vi "reward_behavior_michelle_visjitter_conswinAdapt_enticefx_TSLog.vi"() -> ()   [LabVIEW 2019]
doc: "The myRIO Project template acquires acceleration data from the onboard accelerometer and displays the changes of acceleration values in a waveform chart."
uses:
  <vilib>/myRIO/Common/Instrument Driver Framework/Utilities/typedefs/Generic FPGA Reference.ctl
  <vilib>/myRIO/Common/Instrument Driver Framework/Utilities/typedefs/myRIO v1.0 Reference.ctl
  <vilib>/myRIO/Common/Instrument Driver Framework/Utilities/typedefs/Hardware Version Enum.ctl
  <vilib>/myRIO/Common/Instrument Driver Framework/Utilities/typedefs/myRIO Generic Hardware Reference.ctl
  <vilib>/userdefined/High Color/nirio_resource_hc.ctl
  <vilib>/myRIO/Common/Instrument Driver Framework/Utilities/vis/Is FPGA Ref Available.vi
  <vilib>/myRIO/Common/Instrument Driver Framework/myRIO v1.0/Encoder/typedefs/Encoder Signal Mode.ctl
  <vilib>/myRIO/Common/Instrument Driver Framework/myRIO v1.0/Encoder/typedefs/Encoder Channels Enum.ctl
  <vilib>/myRIO/Instrument Drivers/Onboard IO/Encoder/typedefs/Encoder Reference.ctl
  <vilib>/myRIO/Instrument Drivers/Onboard IO/Encoder/Encoder.lvlib
  <vilib>/myRIO/Instrument Drivers/Onboard IO/Encoder/vis/Read.vi
  <vilib>/myRIO/Common/Instrument Driver Framework/myRIO v1.0/Encoder/typedefs/Encoder Configuration v1.0.ctl
  <vilib>/myRIO/Common/Instrument Driver Framework/myRIO v1.0/Encoder/vis/myRIO v1.1 Open Encoder.vi
  <vilib>/myRIO/Common/Instrument Driver Framework/myRIO v1.0/Encoder/vis/myRIO v1.0 Configure Encoder.vi
  <vilib>/myRIO/Instrument Drivers/Onboard IO/Encoder/vis/myRIO Encoder Open.xnode
  <vilib>/myRIO/Express VI/Onboard IO/Encoder/Encoder Express VI.xnode
  <vilib>/myRIO/Express VI/Onboard IO/DI/DI Express VI.xnode
  <vilib>/myRIO/Instrument Drivers/Onboard IO/DIO/vis/Read.vi
  <vilib>/myRIO/Instrument Drivers/Onboard IO/DIO/DIO.lvlib
  <vilib>/myRIO/Common/Instrument Driver Framework/myRIO v1.0/DIO/typedefs/DIO Channels Enum.ctl
  <vilib>/myRIO/Common/Instrument Driver Framework/myRIO v1.0/DIO/typedefs/DIO Channels List.ctl
  <vilib>/myRIO/Instrument Drivers/Onboard IO/DIO/typedefs/DIO Reference.ctl
  <vilib>/myRIO/Instrument Drivers/Onboard IO/DIO/vis/myRIO DIO Open.xnode
  <vilib>/myRIO/Common/Instrument Driver Framework/myRIO v1.0/DIO/vis/myRIO v1.1 Open DIO.vi
  <vilib>/myRIO/Instrument Drivers/Onboard IO/DIO/vis/Write.vi
  <vilib>/myRIO/Express VI/Onboard IO/DO/DO Express VI.xnode
  <vilib>/Analysis/Matrix/Datatypes/RealMatrix.ctl
  <vilib>/Analysis/Matrix/NI_Matrix.lvlib
panel:
  out "EntTS":dbl[][](array[numeric])
  out "TimeLag":dbl
  out "Lag2":dbl
  out "TestTime":dbl
  out "RewTS":dbl[][](array[numeric])
  out "ConsTS":dbl[][](array[numeric])
  out "LickTS":dbl[][](array[numeric])
  out "ContrastChoice":dbl
  out "Its":i32
  out "BurstCriteria":dbl
  out "LickBurst 2":bool
  out "LickBurst":bool
  out "Enticements":i32
  in  "Entice":bool
  out "Misses":i32
  out "GoAhead":bool
  out "TimeOutDuration":i32
  out "ActiveTime":dbl
  out "ConsumptionGo":bool=TRUE
  out "Consumption_Period":i32
  out "Watch_Display":bool=TRUE
  in  "Give reward":bool
  out "Timings":dbl[](array[numeric])
  out "ISI":dbl
  out "ISI start time":dbl
  out "Time_out":bool=TRUE
  out "Time since lick":dbl
  out "Time of last lick":dbl
  out "Rewarded trials":dbl[](array[numeric])
  out "Rewards":u16
  out "Active Trial":bool
  out "Array temp2":T1
  out "Stimuli Loaded":bool
  out "Stim_ID":dbl[](array[numeric])
  out "Reward_mat":dbl[](array[numeric])
  out "Reward":bool=TRUE
  out "Frame clock":i32
  out "Licks":u32
  out "Lick":bool
  out "Time":dbl
  out "Stop":bool
  in  "Frames to collect":u32
  out "Overflow?":bool
  out "Counter Value":i32
  out "Velocity":dbl
  out "Velocity Plot":dbl[](graph)
  out "Velocity array":dbl[](array[numeric])
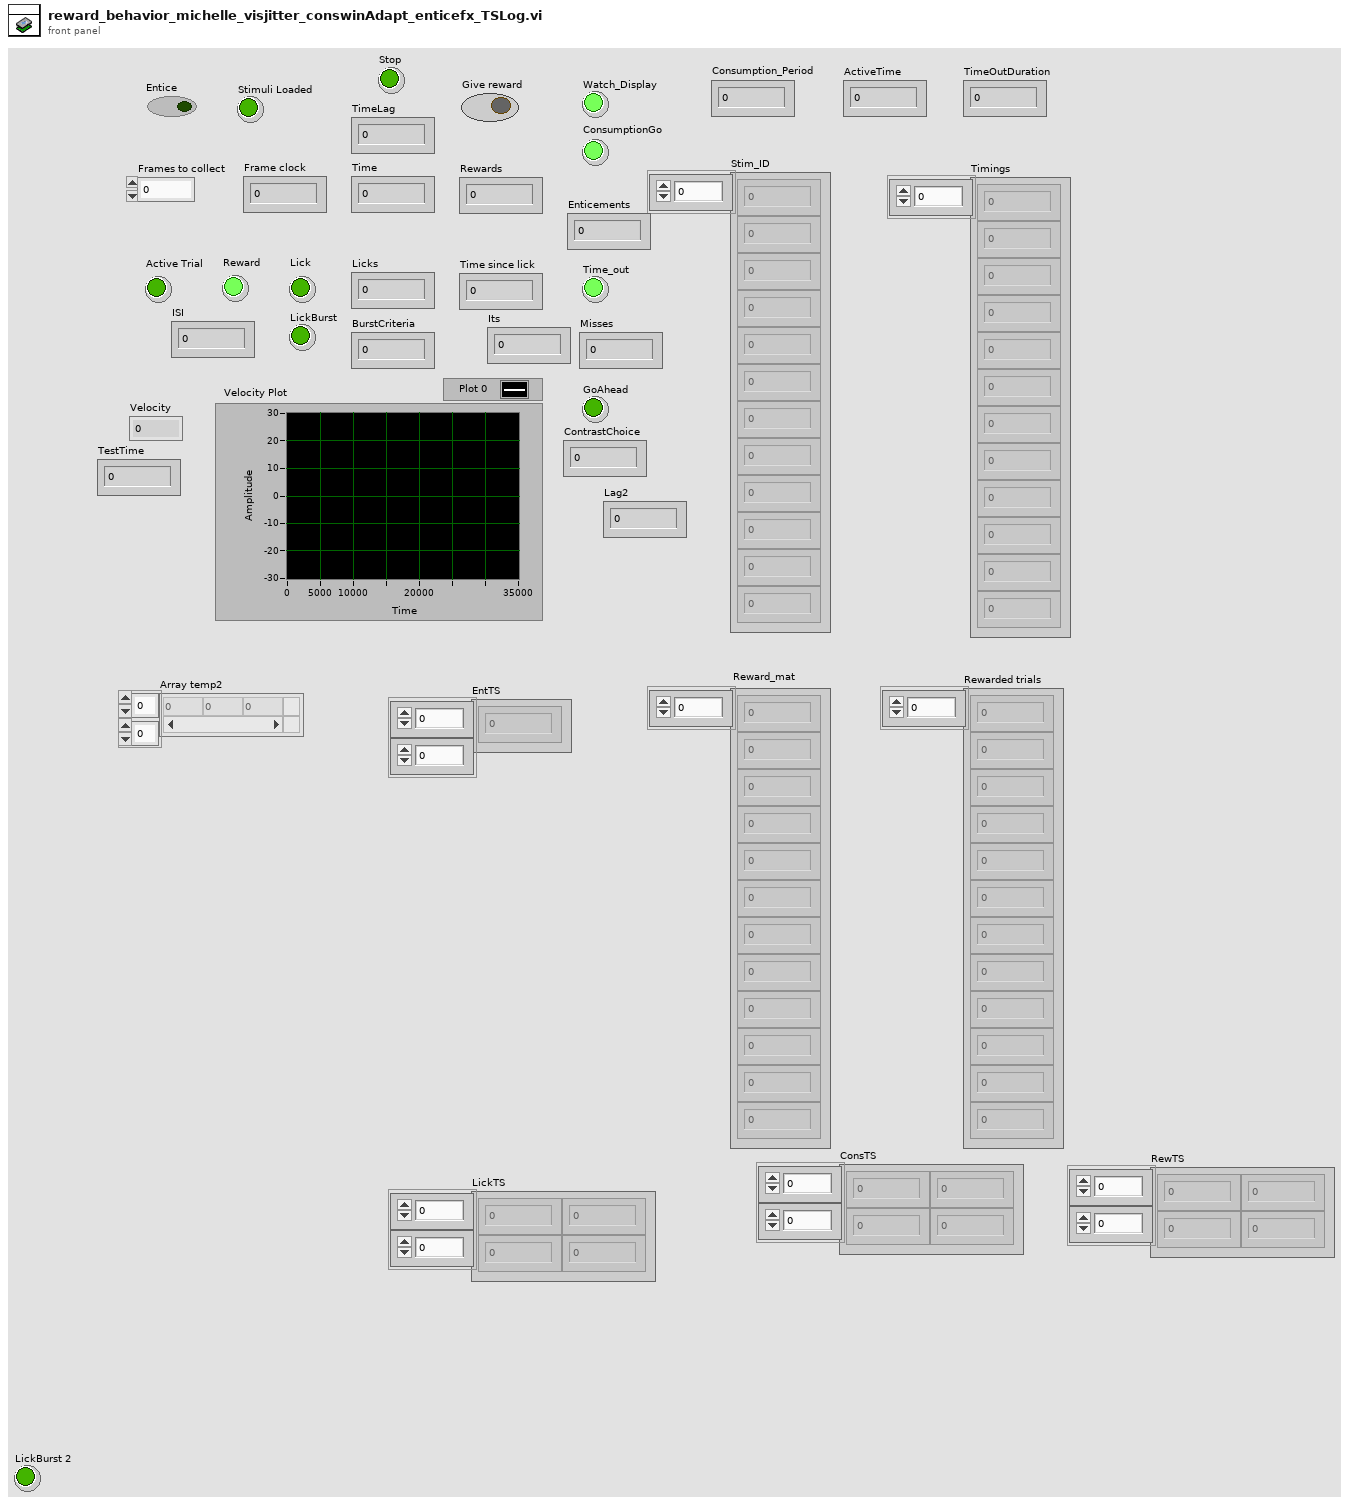
[diagram p1: front panel]
types:
  T1 = typedef "NI_Matrix.lvlib/RealMatrix.ctl" = dbl[][]
  T2 = typedef "Encoder.lvlib/Encoder Reference.ctl" = cluster{"myRIO Reference":T3, "Encoder Channels Enum":T7}
  T3 = typedef "myRIO Generic Hardware Reference.ctl" = cluster{"myRIO Model":T4, "myRIO Hardware Reference":T5}
  T4 = typedef "Hardware Version Enum.ctl" = enum16{"Unknown", "myRIO-1900", "myRIO-1950", "roboRIO", "NI ELVIS RIO CM", "ELVIS III"}
  T5 = typedef "myRIO v1.0 Reference.ctl" = cluster{"Generic FPGA Reference":T6, "Allow multiple opens":bool}
  T6 = typedef "Generic FPGA Reference.ctl" = refnum<k20>
  T7 = typedef "Encoder Channels Enum.ctl" = enum16{"Not Connected", "C/ENC0", "C/ENC1", "A/ENC", "A/ENC0", "A/ENC1", "A/ENC2", "A/ENC3", "A/ENC4", "A/ENC5", "A/ENC6", "A/ENC7", "A/ENC8", "A/ENC9", "B/ENC", "B/ENC0", "B/ENC1", "B/ENC2", "B/ENC3", "B/ENC4", "B/ENC5", "B/ENC6", "B/ENC7", "B/ENC8", "B/ENC9", "DIO/ENC0", "DIO/ENC1", "DIO/ENC2", "DIO/ENC3", "DIO/ENC4"}
  T8 = typedef "Encoder Signal Mode.ctl" = enum16{"Quadrature phase signal", "Step and direction signal"}
  T9 = typedef "nirio_resource_hc.ctl" = tag
  T10 = typedef "DIO.lvlib/DIO Reference.ctl" = cluster{"myRIO Reference":T3, "DIO Channels List":T11}
  T11 = typedef "DIO Channels List.ctl" = T12[]
  T12 = typedef "DIO Channels Enum.ctl" = enum16{"Not Connected", "C/DIO0", "C/DIO1", "C/DIO2", "C/DIO3", "C/DIO4", "C/DIO5", "C/DIO6", "C/DIO7", "A/DIO0", "A/DIO1", "A/DIO2", "A/DIO3", "A/DIO4", "A/DIO5", "A/DIO6", "A/DIO7", "A/DIO8", "A/DIO9", "A/DIO10", "A/DIO11", "A/DIO12", "A/DIO13", "A/DIO14", "A/DIO15", "A/DIO16", "A/DIO17", "A/DIO18", "A/DIO19", "B/DIO0", "B/DIO1", "B/DIO2", "B/DIO3", "B/DIO4", "B/DIO5", "B/DIO6", "B/DIO7", "B/DIO8", "B/DIO9", "B/DIO10", "B/DIO11", "B/DIO12", "B/DIO13", "B/DIO14", "B/DIO15", "B/DIO16", "B/DIO17", "B/DIO18", "B/DIO19", "LED0", "LED1", "LED2", "LED3", "Button0", "DIO/DIO0", "DIO/DIO1", "DIO/DIO2", "DIO/DIO3", "DIO/DIO4", "DIO/DIO5", "DIO/DIO6", "DIO/DIO7", "DIO/DIO8", "DIO/DIO9", "SPI/CS0", "SPI/CS1", "SPI/CS2", "SPI/CS3", "LED RADIO (Green)", "LED RADIO (Red)", "LED COMM (Green)", "LED COMM (Red)", "LED MODE (Green)", "LED MODE (Red)"}
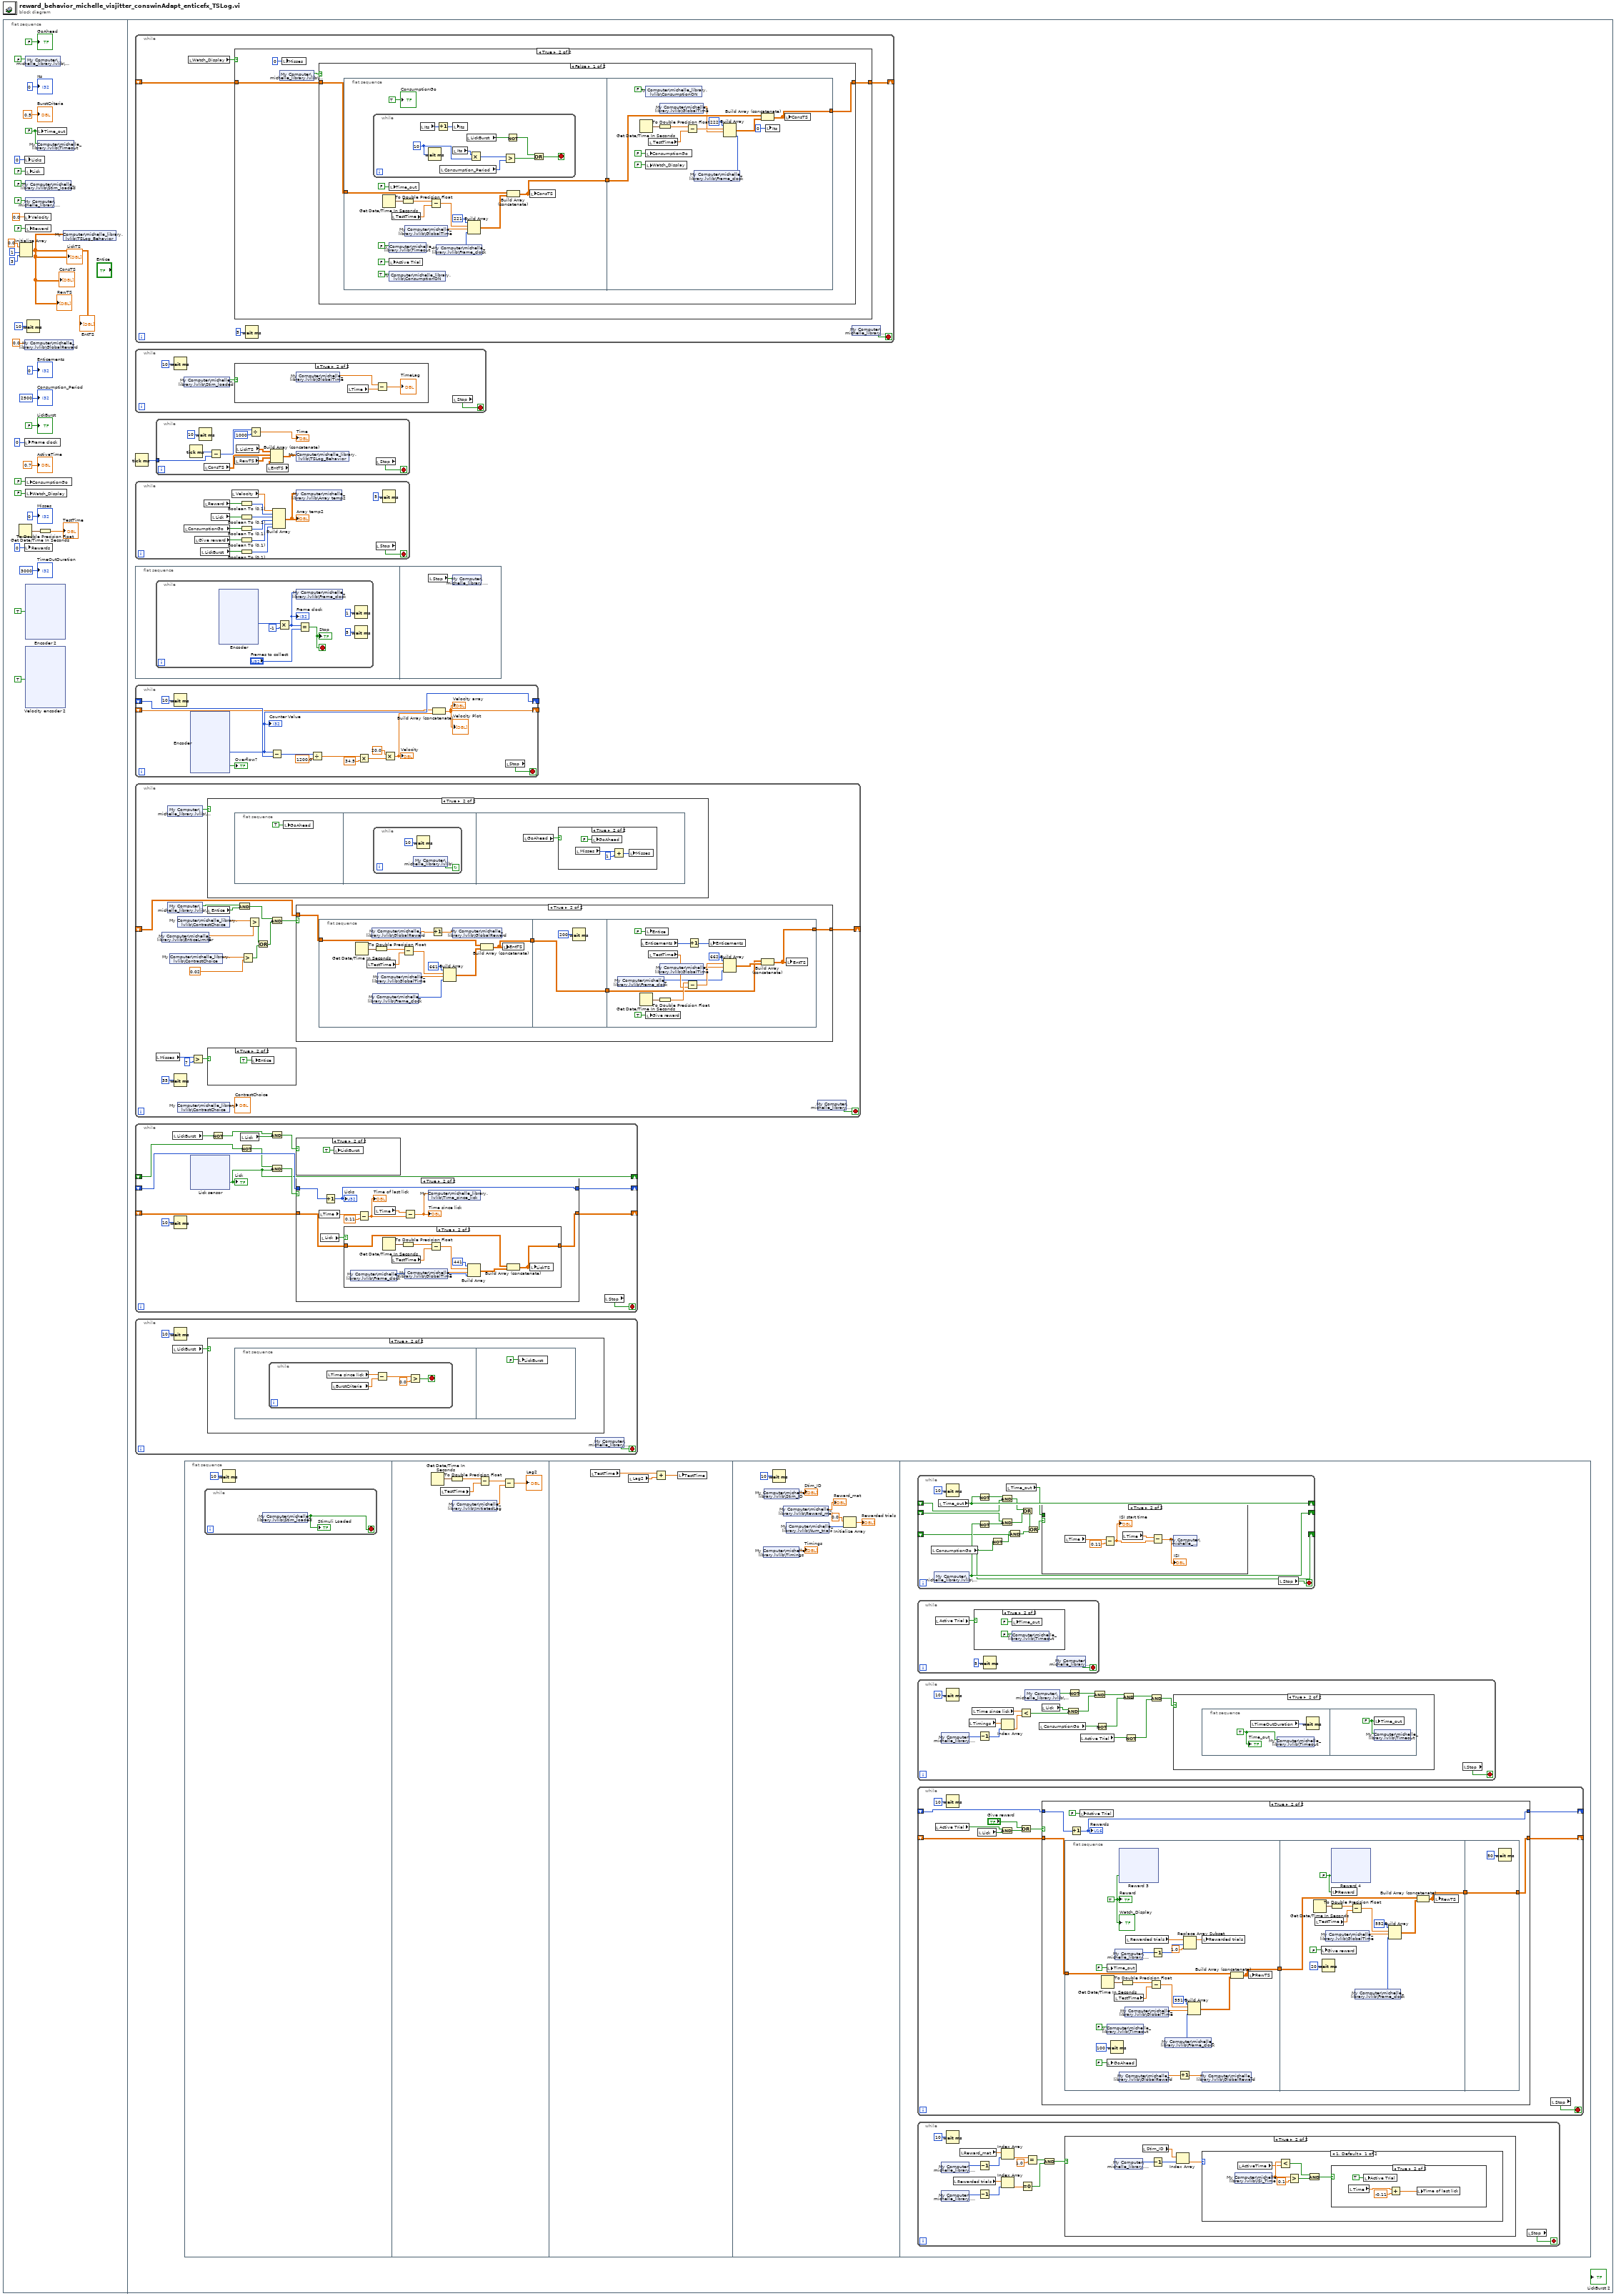
[diagram p0: block diagram]
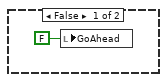
[diagram p6: hidden frame]
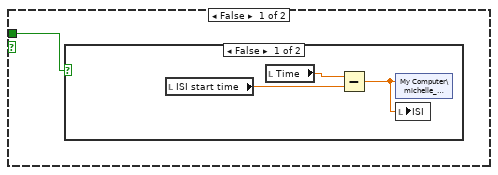
[diagram p12: hidden frame]
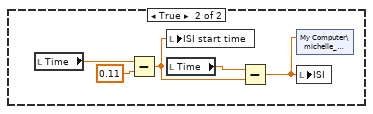
[diagram p13: hidden frame]
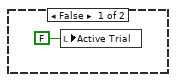
[diagram p14: hidden frame]
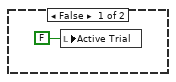
[diagram p15: hidden frame]
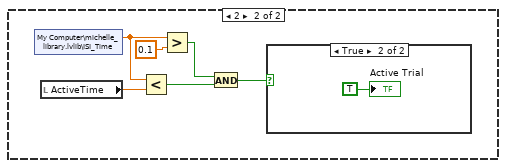
[diagram p16: hidden frame]
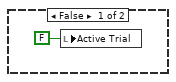
[diagram p17: hidden frame]
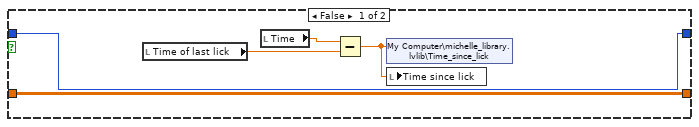
[diagram p20: hidden frame]
diagram:
  n1 = flat-sequence {
    frame #0 {
      w19 = FALSE ("Time_out")
      n2 = Get Date/Time In Seconds() -> (seconds since 1Jan1904=w3:timestamp)
      n3 = Initialize Array(0.0, 1, 3) -> (w1:dbl[][])
      "LickTS" <- w1
      "ConsTS" <- w1
      "RewTS" <- w1
      "EntTS" <- w1
      n4 = local write "Licks"(u32 0 ("Licks")) -> ()
      n5 = local write "Velocity"(0.0 ("Velocity")) -> ()
      n6 = shared-variable "My Computer\\michelle_library.lvlib\\GlobalReward"(0.0) -> ()  [unwired: 1 in, 1 out]
      n7 = local write "Frame clock"(u32 0 ("Frames")) -> ()
      n8 = local write "Rewards"(u16 0 ("Rewards")) -> ()
      n9 = shared-variable "My Computer\\michelle_library.lvlib\\Display"(FALSE ("Display")) -> ()  [unwired: 1 in, 1 out]
      n10 = local write "Lick"(FALSE ("Lick")) -> ()
      n11 = shared-variable "My Computer\\michelle_library.lvlib\\Stim_loaded"(FALSE ("Stim_loaded")) -> ()  [unwired: 1 in, 1 out]
      n12 = shared-variable "My Computer\\michelle_library.lvlib\\Stop"(FALSE ("Stop")) -> ()  [unwired: 1 in, 1 out]
      n13 = local write "Reward"(FALSE ("Give reward")) -> ()
      n14 = local write "ConsumptionGo"(FALSE ("ConsumptionGo")) -> ()
      n15 = local write "Watch_Display"(FALSE ("Watch_Display")) -> ()
      n16 = xnode "Encoder 2"("Reset Counter"=TRUE) -> ()  [unwired: 1 in, 4 out]
      n17 = xnode "Velocity encoder 2"("Reset Counter"=TRUE) -> ()  [unwired: 1 in, 4 out]
      n18 = Wait (ms)(milliseconds to wait=u32 10) -> ()  [unwired: 1 out]
      n19 = local write "Time_out"(w19) -> ()
      n20 = shared-variable "My Computer\\michelle_library.lvlib\\Timeout"(w19) -> ()  [unwired: 1 in, 1 out]
      n21 = To Double Precision Float(number=w3) -> (double precision float=→"TestTime":dbl)
      n22 = shared-variable "My Computer\\michelle_library.lvlib\\TSLog_Behavior"(w1) -> ()  [unwired: 1 in, 1 out]
      "Consumption_Period" <- 2500
      "ActiveTime" <- 0.7
      "TimeOutDuration" <- 3000
      "GoAhead" <- FALSE
      "Misses" <- 0
      "Enticements" <- 0
      "LickBurst" <- FALSE
      "BurstCriteria" <- 0.5
      "Its" <- 0
    }
    frame #1 {
      n23 = while {
        shift-right: [w203] -> _
        shift-left: _ -> [w204]
        stop <- w207 stop-if-true
        n24 = local read "Watch_Display"() -> (w206:bool)
        n25 = case shown="True" w206 {
          tunnel: w204 -> [w208 w210]
          tunnel: [w208 w209] -> w203
          frame False {
          }
          frame True {
            n26 = shared-variable "My Computer\\michelle_library.lvlib\\Display"() -> (w212:bool)  [unwired: 1 in, 1 out]
            n27 = local write "Misses"(0) -> ()
            n28 = case shown="False" w212 {
              tunnel: w210 -> [w215 w255]
              tunnel: [w213 w255] -> w209
              frame False {
                n29 = flat-sequence {
                  tunnel: w215 -> [w219]
                  tunnel: [w218] -> w214
                  tunnel: w214 -> [w245]
                  tunnel: [w244] -> w213
                  frame #0 {
                    n30 = while {
                      stop <- w234 stop-if-true
                      w235 = 10
                      n31 = local read "Its"() -> (w239:i32)
                      n32 = Wait (ms)(milliseconds to wait=w235) -> ()  [unwired: 1 out]
                      n33 = Increment(x=w239) -> (x+1=w238:i32)
                      n34 = local read "Consumption_Period"() -> (w232:i32)
                      n35 = local write "Its"(w238) -> ()
                      n36 = local read "Its"() -> (w236:i32)
                      n37 = local read "LickBurst"() -> (w240:bool)
                      n38 = Multiply(x=w236, y=w235) -> (x*y=w233:i32)
                      n39 = Greater?(x=w233, y=w232) -> (0:w231:bool)
                      n40 = Not(x=w240) -> (.not. x?=w237:bool)
                      n41 = Or(x=w237, y=w231) -> (x .or. y?=w234:bool)
                    }
                    n42 = Get Date/Time In Seconds() -> (seconds since 1Jan1904=w224:timestamp)
                    n43 = local write "Time_out"(FALSE) -> ()
                    n44 = shared-variable "My Computer\\michelle_library.lvlib\\Timeout"(FALSE) -> ()  [unwired: 1 in, 1 out]
                    n45 = local write "Active Trial"(FALSE) -> ()
                    n46 = shared-variable "My Computer\\michelle_library.lvlib\\ConsumptionON"(TRUE) -> ()  [unwired: 1 in, 1 out]
                    n47 = local read "TestTime"() -> (w221:dbl)
                    n48 = To Double Precision Float(number=w224) -> (double precision float=w222:dbl)
                    n49 = shared-variable "My Computer\\michelle_library.lvlib\\GlobalTime"() -> (w217:dbl)  [unwired: 1 in, 1 out]
                    n50 = Subtract(x=w222, y=w221) -> (x-y=w225:dbl)
                    n51 = shared-variable "My Computer\\michelle_library.lvlib\\Frame_clock"() -> (w216:u32)  [unwired: 1 in, 1 out]
                    n52 = Build Array(221, w225, w217, w216) -> (w220:T1)
                    n53 = Build Array (concatenate) ("Build Matrix")(w219, w220) -> (w218:T1)
                    n54 = local write "ConsTS"(w218) -> ()
                    "ConsumptionGo" <- TRUE
                  }
                  frame #1 {
                    n55 = Get Date/Time In Seconds() -> (seconds since 1Jan1904=w249:timestamp)
                    n56 = shared-variable "My Computer\\michelle_library.lvlib\\ConsumptionON"(FALSE) -> ()  [unwired: 1 in, 1 out]
                    n57 = local write "ConsumptionGo"(FALSE ("ConsumptionGo")) -> ()
                    n58 = local write "Watch_Display"(FALSE ("Watch_Display")) -> ()
                    n59 = local read "TestTime"() -> (w246:dbl)
                    n60 = To Double Precision Float(number=w249) -> (double precision float=w247:dbl)
                    n61 = shared-variable "My Computer\\michelle_library.lvlib\\GlobalTime"() -> (w242:dbl)  [unwired: 1 in, 1 out]
                    n62 = Subtract(x=w247, y=w246) -> (x-y=w250:dbl)
                    n63 = shared-variable "My Computer\\michelle_library.lvlib\\Frame_clock"() -> (w241:u32)  [unwired: 1 in, 1 out]
                    n64 = Build Array(222, w250, w242, w241) -> (w243:T1)
                    n65 = Build Array (concatenate) ("Build Matrix")(w245, w243) -> (w244:T1)
                    n66 = local write "Its"(0) -> ()
                    n67 = local write "ConsTS"(w244) -> ()
                  }
                }
              }
              frame True {
              }
            }
          }
        }
        n68 = Wait (ms)(milliseconds to wait=u32 5) -> ()  [unwired: 1 out]
        n69 = shared-variable "My Computer\\michelle_library.lvlib\\Stop"() -> (w207:bool)  [unwired: 1 in, 1 out]
      }
      n70 = while {
        stop <- w126 stop-if-true
        n71 = Wait (ms)(milliseconds to wait=u32 10) -> ()  [unwired: 1 out]
        n72 = shared-variable "My Computer\\michelle_library.lvlib\\Stim_loaded"() -> (w127:bool)  [unwired: 1 in, 1 out]
        n73 = case shown="True" w127 {
          frame False {
          }
          frame True {
            n74 = shared-variable "My Computer\\michelle_library.lvlib\\GlobalTime"() -> (w128:dbl)  [unwired: 1 in, 1 out]
            n75 = local read "Time"() -> (w129:dbl)
            n76 = Subtract(x=w128, y=w129) -> (x-y=→"TimeLag":dbl)
          }
        }
        n77 = local read "Stop"() -> (w126:bool)
      }
      n78 = Tick Count (ms)() -> (millisecond timer value=w124:u32)
      n79 = while {
        stop <- w263 stop-if-true
        n80 = local read "ConsumptionGo"() -> (w261:bool)
        n81 = local read "Give reward"() -> (w260:bool)
        n82 = local read "LickBurst"() -> (w257:bool)
        n83 = local read "Reward"() -> (w268:bool)
        n84 = local read "Lick"() -> (w269:bool)
        n85 = local read "Velocity"() -> (w267:dbl)
        n86 = Boolean To (0,1)(Boolean=w268) -> (0, 1=w266:i16)
        n87 = Boolean To (0,1)(Boolean=w269) -> (0, 1=w265:i16)
        n88 = Boolean To (0,1)(Boolean=w261) -> (0, 1=w259:i16)
        n89 = Boolean To (0,1)(Boolean=w260) -> (0, 1=w258:i16)
        n90 = Boolean To (0,1)(Boolean=w257) -> (0, 1=w256:i16)
        n91 = Build Array(w267, w266, w265, w259, w258, w256) -> (w262:T1)
        "Array temp2" <- w262
        n92 = shared-variable "My Computer\\michelle_library.lvlib\\Array temp2"(w262) -> ()  [unwired: 1 in, 1 out]
        n93 = local read "Stop"() -> (w263:bool)
        n94 = Wait (ms)(milliseconds to wait=u32 5) -> ()  [unwired: 1 out]
      }
      n95 = flat-sequence {
        frame #0 {
          n96 = while {
            stop <- w512 stop-if-true
            n97 = xnode "Encoder"() -> ("Counter Value"=w516:i32)  [unwired: 2 in, 3 out]
            n98 = Multiply(x=w516, y=-1) -> (x*y=w511:i32)
            "Frame clock" <- w511
            n99 = shared-variable "My Computer\\michelle_library.lvlib\\Frame_clock"(w511) -> ()  [unwired: 1 in, 1 out]
            n100 = Equal?(x=w511, y="Frames to collect") -> (x = y?=w512:bool)
            "Stop" <- w512
            n101 = Wait (ms)(milliseconds to wait=u32 1) -> ()  [unwired: 1 out]
            n102 = Wait (ms)(milliseconds to wait=u32 5) -> ()  [unwired: 1 out]
          }
        }
        frame #1 {
          n103 = local read "Stop"() -> (w564:bool)
          n104 = shared-variable "My Computer\\michelle_library.lvlib\\Stop"(w564) -> ()  [unwired: 1 in, 1 out]
        }
      }
      n105 = while {
        shift-right: [w651] -> _
        shift-left: _ -> [w652]
        shift-right: [w643] -> _
        shift-left: _ -> [w642]
        stop <- w641 stop-if-true
        n106 = Wait (ms)(milliseconds to wait=u32 10) -> ()  [unwired: 1 out]
        n107 = xnode "Encoder"() -> ("Counter Value"=w651:i32, "Overflow?"=→"Overflow?":bool)  [unwired: 2 in, 2 out]
        "Counter Value" <- w651
        n108 = Subtract(x=w651, y=w652) -> (x-y=w644:i32)
        n109 = Divide(x=w644, y=1200.0 ("600")) -> (x/y=w649:dbl)
        n110 = Multiply(x=w649, y=34.5) -> (x*y=w647:dbl)
        n111 = Multiply(x=20.0, y=w647) -> (x*y=w645:dbl)
        "Velocity" <- w645
        n112 = Build Array (concatenate)(w642, w645) -> (w643:dbl[])
        "Velocity Plot" <- w643
        "Velocity array" <- w643
        n113 = local read "Stop"() -> (w641:bool)
      }
      n114 = while {
        shift-right: [w146] -> _
        shift-left: _ -> [w147]
        stop <- w159 stop-if-true
        n115 = local read "Misses"() -> (w157:i32)
        n116 = shared-variable "My Computer\\michelle_library.lvlib\\EnticeLimiter"() -> (w145:dbl)  [unwired: 1 in, 1 out]
        n117 = shared-variable "My Computer\\michelle_library.lvlib\\Display"() -> (w158:bool)  [unwired: 1 in, 1 out]
        n118 = shared-variable "My Computer\\michelle_library.lvlib\\Display"() -> (w154:bool)  [unwired: 1 in, 1 out]
        n119 = shared-variable "My Computer\\michelle_library.lvlib\\ContrastChoice"() -> (w141:dbl)  [unwired: 1 in, 1 out]
        n120 = Wait (ms)(milliseconds to wait=35) -> ()  [unwired: 1 out]
        n121 = shared-variable "My Computer\\michelle_library.lvlib\\ContrastChoice"() -> (w150:dbl)  [unwired: 1 in, 1 out]
        n122 = shared-variable "My Computer\\michelle_library.lvlib\\ContrastChoice"() -> (→"ContrastChoice":dbl)  [unwired: 1 in, 1 out]
        n123 = Greater?(x=w157, y=7) -> (0:w155:bool)
        n124 = case shown="True" w158 {
          frame False {
            n125 = local write "GoAhead"(FALSE) -> ()
          }
          frame True {
            n126 = flat-sequence {
              frame #0 {
                n127 = local write "GoAhead"(TRUE) -> ()
              }
              frame #1 {
                n128 = while {
                  stop <- w197 continue-if-true
                  n129 = shared-variable "My Computer\\michelle_library.lvlib\\Display"() -> (w197:bool)  [unwired: 1 in, 1 out]
                  n130 = Wait (ms)(milliseconds to wait=10) -> ()  [unwired: 1 out]
                }
              }
              frame #2 {
                n131 = local read "GoAhead"() -> (w198:bool)
                n132 = case shown="True" w198 {
                  frame False {
                  }
                  frame True {
                    n133 = local read "Misses"() -> (w202:i32)
                    n134 = local write "GoAhead"(FALSE) -> ()
                    n135 = Add(x=w202, y=1) -> (x+y=w200:i32)
                    n136 = local write "Misses"(w200) -> ()
                  }
                }
              }
            }
          }
        }
        n137 = local read "Entice"() -> (w153:bool)
        n138 = case shown="True" w155 {
          frame False {
          }
          frame True {
            n139 = local write "Entice"(TRUE) -> ()
          }
        }
        n140 = And(x=w154, y=w153) -> (x .and. y?=w151:bool)
        n141 = Greater?(x=w141, y=0.02) -> (0:w142:bool)
        n142 = Greater?(x=w150, y=w145) -> (0:w143:bool)
        n143 = Or(x=w143, y=w142) -> (x .or. y?=w144:bool)
        n144 = And(x=w151, y=w144) -> (x .and. y?=w149:bool)
        n145 = case shown="True" w149 {
          tunnel: w147 -> [w160 w164]
          tunnel: [w160 w161] -> w146
          frame False {
          }
          frame True {
            n146 = flat-sequence {
              tunnel: w164 -> [w167]
              tunnel: [w166] -> w163
              tunnel: w163 -> [w177]
              tunnel: [w177] -> w162
              tunnel: w162 -> [w181]
              tunnel: [w180] -> w161
              frame #0 {
                n147 = Get Date/Time In Seconds() -> (seconds since 1Jan1904=w174:timestamp)
                n148 = local read "TestTime"() -> (w169:dbl)
                n149 = shared-variable "My Computer\\michelle_library.lvlib\\GlobalReward"() -> (w176:dbl)  [unwired: 1 in, 1 out]
                n150 = shared-variable "My Computer\\michelle_library.lvlib\\Frame_clock"() -> (w165:u32)  [unwired: 1 in, 1 out]
                n151 = To Double Precision Float(number=w174) -> (double precision float=w173:dbl)
                n152 = shared-variable "My Computer\\michelle_library.lvlib\\GlobalTime"() -> (w168:dbl)  [unwired: 1 in, 1 out]
                n153 = Subtract(x=w173, y=w169) -> (x-y=w172:dbl)
                n154 = Increment(x=w176) -> (x+1=w175:dbl)
                n155 = Build Array(661, w172, w168, w165) -> (w171:T1)
                n156 = shared-variable "My Computer\\michelle_library.lvlib\\GlobalReward"(w175) -> ()  [unwired: 1 in, 1 out]
                n157 = Build Array (concatenate) ("Build Matrix")(w167, w171) -> (w166:T1)
                n158 = local write "EntTS"(w166) -> ()
              }
              frame #1 {
                n159 = Wait (ms)(milliseconds to wait=200) -> ()  [unwired: 1 out]
              }
              frame #2 {
                n160 = shared-variable "My Computer\\michelle_library.lvlib\\Frame_clock"() -> (w179:u32)  [unwired: 1 in, 1 out]
                n161 = Get Date/Time In Seconds() -> (seconds since 1Jan1904=w188:timestamp)
                n162 = local read "Enticements"() -> (w190:i32)
                n163 = local write "Entice"(FALSE) -> ()
                n164 = local write "Give reward"(TRUE) -> ()
                n165 = local read "TestTime"() -> (w182:dbl)
                n166 = To Double Precision Float(number=w188) -> (double precision float=w187:dbl)
                n167 = shared-variable "My Computer\\michelle_library.lvlib\\GlobalTime"() -> (w183:dbl)  [unwired: 1 in, 1 out]
                n168 = Subtract(x=w187, y=w182) -> (x-y=w186:dbl)
                n169 = Increment(x=w190) -> (x+1=w189:i32)
                n170 = local write "Enticements"(w189) -> ()
                n171 = Build Array(662, w186, w183, w179) -> (w185:T1)
                n172 = Build Array (concatenate) ("Build Matrix")(w181, w185) -> (w180:T1)
                n173 = local write "EntTS"(w180) -> ()
              }
            }
          }
        }
        n174 = shared-variable "My Computer\\michelle_library.lvlib\\Stop"() -> (w159:bool)  [unwired: 1 in, 1 out]
      }
      n175 = while {
        shift-right: [w577] -> _
        shift-left: _ -> [w576]
        shift-right: [w571] -> _
        shift-left: _ -> [w574]
        shift-right: [w565] -> _
        shift-left: _ -> [w566]
        stop <- w575 stop-if-true
        n176 = local read "LickBurst"() -> (w568:bool)
        n177 = Wait (ms)(milliseconds to wait=u32 10) -> ()  [unwired: 1 out]
        n178 = xnode "Lick sensor"() -> ("C/DIO1 (DIO1)"=w571:bool)  [unwired: 1 in, 1 out]
        "Lick" <- w571
        n179 = Not(x=w568) -> (.not. x?=w567:bool)
        n180 = Not(x=w574) -> (.not. x?=w573:bool)
        n181 = local read "Lick"() -> (w569:bool)
        n182 = And(x=w567, y=w569) -> (x .and. y?=w570:bool)
        n183 = And(x=w573, y=w571) -> (x .and. y?=w572:bool)
        n184 = case shown="True" w570 {
          frame False {
          }
          frame True {
            n185 = local write "LickBurst"(TRUE) -> ()
          }
        }
        n186 = case shown="True" w572 {
          tunnel: [w584 w594] -> w577
          tunnel: w576 -> [w584 w593]
          tunnel: w566 -> [w580 w585]
          tunnel: [w580 w587] -> w565
          frame False {
            n187 = local read "Time of last lick"() -> (w582:dbl)
            n188 = local read "Time"() -> (w583:dbl)
            n189 = Subtract(x=w583, y=w582) -> (x-y=w581:dbl)
            n190 = shared-variable "My Computer\\michelle_library.lvlib\\Time_since_lick"(w581) -> ()  [unwired: 1 in, 1 out]
            n191 = local write "Time since lick"(w581) -> ()
          }
          frame True {
            n192 = local read "Time"() -> (w590:dbl)
            n193 = local read "Lick"() -> (w586:bool)
            n194 = Increment(x=w593) -> (x+1=w594:u32)
            "Licks" <- w594
            n195 = case shown="True" w586 {
              tunnel: w585 -> [w595 w601]
              tunnel: [w595 w600] -> w587
              frame False {
              }
              frame True {
                n196 = shared-variable "My Computer\\michelle_library.lvlib\\Frame_clock"() -> (w596:u32)  [unwired: 1 in, 1 out]
                n197 = Get Date/Time In Seconds() -> (seconds since 1Jan1904=w603:timestamp)
                n198 = local read "TestTime"() -> (w598:dbl)
                n199 = To Double Precision Float(number=w603) -> (double precision float=w599:dbl)
                n200 = shared-variable "My Computer\\michelle_library.lvlib\\GlobalTime"() -> (w597:dbl)  [unwired: 1 in, 1 out]
                n201 = Subtract(x=w599, y=w598) -> (x-y=w604:dbl)
                n202 = Build Array(441, w604, w597, w596) -> (w605:T1)
                n203 = Build Array (concatenate) ("Build Matrix")(w601, w605) -> (w600:T1)
                n204 = local write "LickTS"(w600) -> ()
              }
            }
            n205 = Subtract(x=w590, y=0.11) -> (x-y=w588:dbl)
            "Time of last lick" <- w588
            n206 = local read "Time"() -> (w592:dbl)
            n207 = Subtract(x=w592, y=w588) -> (x-y=w591:dbl)
            "Time since lick" <- w591
            n208 = shared-variable "My Computer\\michelle_library.lvlib\\Time_since_lick"(w591) -> ()  [unwired: 1 in, 1 out]
          }
        }
        n209 = local read "Stop"() -> (w575:bool)
      }
      n210 = while {
        stop <- w133 stop-if-true
        n211 = local read "LickBurst"() -> (w131:bool)
        n212 = Wait (ms)(milliseconds to wait=u32 10) -> ()  [unwired: 1 out]
        n213 = case shown="True" w131 {
          frame False {
          }
          frame True {
            n214 = flat-sequence {
              frame #0 {
                n215 = while {
                  stop <- w136 stop-if-true
                  n216 = local read "Time since lick"() -> (w137:dbl)
                  n217 = local read "BurstCriteria"() -> (w138:dbl)
                  n218 = Subtract(x=w137, y=w138) -> (x-y=w134:dbl)
                  n219 = Greater?(x=w134, y=0.0) -> (0:w136:bool)
                }
              }
              frame #1 {
                n220 = local write "LickBurst"(FALSE) -> ()
              }
            }
          }
        }
        n221 = shared-variable "My Computer\\michelle_library.lvlib\\Stop"() -> (w133:bool)  [unwired: 1 in, 1 out]
      }
      n222 = while {
        tunnel: w124 -> [w711]
        stop <- w709 stop-if-true
        n223 = Tick Count (ms)() -> (millisecond timer value=w712:u32)
        n224 = Wait (ms)(milliseconds to wait=u32 10) -> ()  [unwired: 1 out]
        n225 = local read "ConsTS"() -> (w704:dbl[][])
        n226 = Subtract(x=w712, y=w711) -> (x-y=w708:u32)
        n227 = local read "RewTS"() -> (w703:dbl[][])
        n228 = local read "LickTS"() -> (w705:dbl[][])
        n229 = Divide(x=w708, y=u32 1000) -> (x/y=→"Time":dbl)
        n230 = local read "EntTS"() -> (w701:dbl[][])
        n231 = Build Array (concatenate) ("Build Matrix")(w705, w704, w703, w701) -> (w702:T1)
        n232 = shared-variable "My Computer\\michelle_library.lvlib\\TSLog_Behavior"(w702) -> ()  [unwired: 1 in, 1 out]
        n233 = local read "Stop"() -> (w709:bool)
      }
      n234 = flat-sequence {
        frame #0 {
          n235 = while {
            stop <- w271 stop-if-true
            n236 = shared-variable "My Computer\\michelle_library.lvlib\\Stim_loaded"() -> (w271:bool)  [unwired: 1 in, 1 out]
            "Stimuli Loaded" <- w271
          }
          n237 = Wait (ms)(milliseconds to wait=u32 10) -> ()  [unwired: 1 out]
        }
        frame #1 {
          n238 = Get Date/Time In Seconds() -> (seconds since 1Jan1904=w277:timestamp)
          n239 = local read "TestTime"() -> (w276:dbl)
          n240 = To Double Precision Float(number=w277) -> (double precision float=w275:dbl)
          n241 = shared-variable "My Computer\\michelle_library.lvlib\\InitiatedLag"() -> (w274:dbl)  [unwired: 1 in, 1 out]
          n242 = Subtract(x=w275, y=w276) -> (x-y=w272:dbl)
          n243 = Subtract(x=w272, y=w274) -> (x-y=→"Lag2":dbl)
        }
        frame #2 {
          n244 = local read "TestTime"() -> (w278:dbl)
          n245 = local read "Lag2"() -> (w279:dbl)
          n246 = Add(x=w278, y=w279) -> (x+y=w280:dbl)
          n247 = local write "TestTime"(w280) -> ()
        }
        frame #3 {
          n248 = shared-variable "My Computer\\michelle_library.lvlib\\Timings"() -> (→"Timings":dbl[])  [unwired: 1 in, 1 out]
          n249 = shared-variable "My Computer\\michelle_library.lvlib\\Stim_ID"() -> (→"Stim_ID":dbl[])  [unwired: 1 in, 1 out]
          n250 = Wait (ms)(milliseconds to wait=u32 10) -> ()  [unwired: 1 out]
          n251 = shared-variable "My Computer\\michelle_library.lvlib\\Reward_mat"() -> (→"Reward_mat":dbl[])  [unwired: 1 in, 1 out]
          n252 = shared-variable "My Computer\\michelle_library.lvlib\\Num_trials"() -> (w284:u32)  [unwired: 1 in, 1 out]
          n253 = Initialize Array(0.0 ("element"), w284) -> (→"Rewarded trials":dbl[])
        }
        frame #4 {
          n254 = while {
            shift-right: [w330] -> _
            shift-left: _ -> [w328]
            shift-right: [w326] -> _
            shift-left: _ -> [w325]
            shift-right: [w320] -> _
            shift-left: _ -> [w318]
            stop <- w331 stop-if-true
            n255 = local read "ConsumptionGo"() -> (w320:bool)
            n256 = shared-variable "My Computer\\michelle_library.lvlib\\Display"() -> (w326:bool)  [unwired: 1 in, 1 out]
            n257 = local read "Time_out"() -> (w330:bool)
            n258 = Wait (ms)(milliseconds to wait=u32 10) -> ()  [unwired: 1 out]
            n259 = Not(x=w330) -> (.not. x?=w329:bool)
            n260 = Not(x=w326) -> (.not. x?=w324:bool)
            n261 = Not(x=w320) -> (.not. x?=w321:bool)
            n262 = And(x=w329, y=w328) -> (x .and. y?=w323:bool)
            n263 = And(x=w325, y=w324) -> (x .and. y?=w319:bool)
            n264 = local read "Time_out"() -> (w327:bool)
            n265 = And(x=w318, y=w321) -> (x .and. y?=w317:bool)
            n266 = Or(x=w323, y=w319) -> (x .or. y?=w316:bool)
            n267 = Or(x=w316, y=w317) -> (x .or. y?=w315:bool)
            n268 = case shown="True" w315 {
              tunnel: w327 -> [w332 _]
              frame False {
                n269 = case shown="False" w332 {
                  frame False {
                    n270 = local read "ISI start time"() -> (w335:dbl)
                    n271 = local read "Time"() -> (w334:dbl)
                    n272 = Subtract(x=w334, y=w335) -> (x-y=w333:dbl)
                    n273 = shared-variable "My Computer\\michelle_library.lvlib\\ISI"(w333) -> ()  [unwired: 1 in, 1 out]
                    n274 = local write "ISI"(w333) -> ()
                  }
                  frame True {
                    n275 = local read "Time"() -> (w340:dbl)
                    n276 = Subtract(x=w340, y=0.11) -> (x-y=w337:dbl)
                    n277 = local write "ISI start time"(w337) -> ()
                    n278 = local read "Time"() -> (w338:dbl)
                    n279 = Subtract(x=w338, y=w337) -> (x-y=w336:dbl)
                    n280 = shared-variable "My Computer\\michelle_library.lvlib\\ISI"(w336) -> ()  [unwired: 1 in, 1 out]
                    n281 = local write "ISI"(w336) -> ()
                  }
                }
              }
              frame True {
                n282 = local read "Time"() -> (w345:dbl)
                n283 = Subtract(x=w345, y=0.11) -> (x-y=w342:dbl)
                "ISI start time" <- w342
                n284 = local read "Time"() -> (w343:dbl)
                n285 = Subtract(x=w343, y=w342) -> (x-y=w341:dbl)
                "ISI" <- w341
                n286 = shared-variable "My Computer\\michelle_library.lvlib\\ISI"(w341) -> ()  [unwired: 1 in, 1 out]
              }
            }
            n287 = local read "Stop"() -> (w331:bool)
          }
          n288 = while {
            stop <- w290 stop-if-true
            n289 = local read "Active Trial"() -> (w289:bool)
            n290 = case shown="True" w289 {
              frame False {
              }
              frame True {
                n291 = local write "Time_out"(FALSE) -> ()
                n292 = shared-variable "My Computer\\michelle_library.lvlib\\Timeout"(FALSE) -> ()  [unwired: 1 in, 1 out]
              }
            }
            n293 = Wait (ms)(milliseconds to wait=5) -> ()  [unwired: 1 out]
            n294 = shared-variable "My Computer\\michelle_library.lvlib\\Stop"() -> (w290:bool)  [unwired: 1 in, 1 out]
          }
          n295 = while {
            stop <- w311 stop-if-true
            n296 = shared-variable "My Computer\\michelle_library.lvlib\\Trial"() -> (w301:u32)  [unwired: 1 in, 1 out]
            n297 = Wait (ms)(milliseconds to wait=u32 10) -> ()  [unwired: 1 out]
            n298 = local read "Timings"() -> (w303:dbl[])
            n299 = local read "Time since lick"() -> (w310:dbl)
            n300 = Decrement(x=w301) -> (x-1=w300:u32)
            n301 = Index Array(array=w303, index=w300) -> (element=w302:dbl)
            n302 = Less?(x=w310, y=w302) -> (x < y?=w309:bool)
            n303 = shared-variable "My Computer\\michelle_library.lvlib\\Display"() -> (w306:bool)  [unwired: 1 in, 1 out]
            n304 = local read "ConsumptionGo"() -> (w298:bool)
            n305 = local read "Lick"() -> (w308:bool)
            n306 = And(x=w308, y=w309) -> (x .and. y?=w304:bool)
            n307 = Not(x=w306) -> (.not. x?=w305:bool)
            n308 = local read "Active Trial"() -> (w293:bool)
            n309 = And(x=w305, y=w304) -> (x .and. y?=w297:bool)
            n310 = Not(x=w298) -> (.not. x?=w299:bool)
            n311 = And(x=w297, y=w299) -> (x .and. y?=w295:bool)
            n312 = Not(x=w293) -> (.not. x?=w296:bool)
            n313 = And(x=w295, y=w296) -> (x .and. y?=w294:bool)
            n314 = case shown="True" w294 {
              frame False {
              }
              frame True {
                n315 = flat-sequence {
                  frame #0 {
                    w313 = TRUE
                    n316 = local read "TimeOutDuration"() -> (w312:i32)
                    n317 = shared-variable "My Computer\\michelle_library.lvlib\\Timeout"(w313) -> ()  [unwired: 1 in, 1 out]
                    n318 = Wait (ms)(milliseconds to wait=w312) -> ()  [unwired: 1 out]
                    "Time_out" <- w313
                  }
                  frame #1 {
                    w314 = FALSE ("Timeout")
                    n319 = local write "Time_out"(w314) -> ()
                    n320 = shared-variable "My Computer\\michelle_library.lvlib\\Timeout"(w314) -> ()  [unwired: 1 in, 1 out]
                  }
                }
              }
            }
            n321 = local read "Stop"() -> (w311:bool)
          }
          n322 = while {
            shift-right: [w392] -> _
            shift-left: _ -> [w391]
            shift-right: [w384] -> _
            shift-left: _ -> [w385]
            stop <- w394 stop-if-true
            n323 = local read "Active Trial"() -> (w389:bool)
            n324 = Wait (ms)(milliseconds to wait=u32 10) -> ()  [unwired: 1 out]
            n325 = local read "Lick"() -> (w390:bool)
            n326 = And(x=w389, y=w390) -> (x .and. y?=w388:bool)
            n327 = Or(x="Give reward", y=w388) -> (x .or. y?=w387:bool)
            n328 = case shown="True" w387 {
              tunnel: [w396 w403] -> w392
              tunnel: w391 -> [w396 w402]
              tunnel: w385 -> [w395 w400]
              tunnel: [w395 w399] -> w384
              frame False {
              }
              frame True {
                n329 = flat-sequence {
                  tunnel: w400 -> [w409]
                  tunnel: [w406] -> w397
                  tunnel: [w465] -> w398
                  tunnel: w397 -> [w463]
                  tunnel: [w509] -> w399
                  tunnel: w398 -> [w509]
                  frame #0 {
                    w424 = TRUE ("C/DIO0 (DIO0)")
                    n330 = Get Date/Time In Seconds() -> (seconds since 1Jan1904=w413:timestamp)
                    n331 = local write "Time_out"(FALSE) -> ()
                    n332 = shared-variable "My Computer\\michelle_library.lvlib\\Timeout"(FALSE) -> ()  [unwired: 1 in, 1 out]
                    n333 = local write "GoAhead"(FALSE) -> ()
                    n334 = Wait (ms)(milliseconds to wait=u32 100) -> ()  [unwired: 1 out]
                    n335 = local read "TestTime"() -> (w407:dbl)
                    n336 = shared-variable "My Computer\\michelle_library.lvlib\\Trial"() -> (w423:u32)  [unwired: 1 in, 1 out]
                    n337 = xnode "Reward 3"("C/DIO0 (DIO0)"=w424) -> ()  [unwired: 1 in, 1 out]
                    n338 = shared-variable "My Computer\\michelle_library.lvlib\\GlobalReward"() -> (w415:dbl)  [unwired: 1 in, 1 out]
                    n339 = To Double Precision Float(number=w413) -> (double precision float=w412:dbl)
                    n340 = shared-variable "My Computer\\michelle_library.lvlib\\GlobalTime"() -> (w405:dbl)  [unwired: 1 in, 1 out]
                    n341 = local read "Rewarded trials"() -> (w421:dbl[])
                    n342 = Subtract(x=w412, y=w407) -> (x-y=w411:dbl)
                    n343 = Decrement(x=w423) -> (x-1=w422:u32)
                    n344 = shared-variable "My Computer\\michelle_library.lvlib\\Frame_clock"() -> (w404:u32)  [unwired: 1 in, 1 out]
                    n345 = Increment(x=w415) -> (x+1=w414:dbl)
                    n346 = Replace Array Subset(array=w421, new element=1.0 ("new element/subarray"), index=w422) -> (w419:dbl[])
                    n347 = Build Array(551, w411, w405, w404) -> (w410:T1)
                    n348 = local write "Rewarded trials"(w419) -> ()
                    n349 = shared-variable "My Computer\\michelle_library.lvlib\\GlobalReward"(w414) -> ()  [unwired: 1 in, 1 out]
                    n350 = Build Array (concatenate) ("Build Matrix")(w409, w410) -> (w406:T1)
                    n351 = local write "RewTS"(w406) -> ()
                    "Reward" <- w424
                    "Watch_Display" <- w424
                  }
                  frame #1 {
                    w473 = FALSE ("C/DIO0 (DIO0)")
                    n352 = Get Date/Time In Seconds() -> (seconds since 1Jan1904=w470:timestamp)
                    n353 = local read "TestTime"() -> (w464:dbl)
                    n354 = local write "Give reward"(FALSE ("Give reward")) -> ()
                    n355 = Wait (ms)(milliseconds to wait=u32 20) -> ()  [unwired: 1 out]
                    n356 = shared-variable "My Computer\\michelle_library.lvlib\\GlobalTime"() -> (w462:dbl)  [unwired: 1 in, 1 out]
                    n357 = To Double Precision Float(number=w470) -> (double precision float=w469:dbl)
                    n358 = xnode "Reward 4"("C/DIO0 (DIO0)"=w473) -> ()  [unwired: 1 in, 1 out]
                    n359 = local write "Reward"(w473) -> ()
                    n360 = Subtract(x=w469, y=w464) -> (x-y=w468:dbl)
                    n361 = shared-variable "My Computer\\michelle_library.lvlib\\Frame_clock"() -> (w461:u32)  [unwired: 1 in, 1 out]
                    n362 = Build Array(552, w468, w462, w461) -> (w466:T1)
                    n363 = Build Array (concatenate) ("Build Matrix")(w463, w466) -> (w465:T1)
                    n364 = local write "RewTS"(w465) -> ()
                  }
                  frame #2 {
                    n365 = Wait (ms)(milliseconds to wait=u32 50) -> ()  [unwired: 1 out]
                  }
                }
                n366 = Increment(x=w402) -> (x+1=w403:u16)
                "Rewards" <- w403
                n367 = local write "Active Trial"(FALSE ("Active Trial")) -> ()
              }
            }
            n368 = local read "Stop"() -> (w394:bool)
          }
          n369 = while {
            stop <- w359 stop-if-true
            n370 = shared-variable "My Computer\\michelle_library.lvlib\\Trial"() -> (w355:u32)  [unwired: 1 in, 1 out]
            n371 = shared-variable "My Computer\\michelle_library.lvlib\\Trial"() -> (w351:u32)  [unwired: 1 in, 1 out]
            n372 = Wait (ms)(milliseconds to wait=u32 10) -> ()  [unwired: 1 out]
            n373 = local read "Rewarded trials"() -> (w352:dbl[])
            n374 = local read "Reward_mat"() -> (w354:dbl[])
            n375 = Decrement(x=w355) -> (x-1=w356:u32)
            n376 = Decrement(x=w351) -> (x-1=w350:u32)
            n377 = Index Array(array=w354, index=w356) -> (element=w357:dbl)
            n378 = Index Array(array=w352, index=w350) -> (element=w349:dbl)
            n379 = Equal To 0?(x=w349) -> (x = 0?=w348:bool)
            n380 = Equal?(x=w357, y=1.0) -> (x = y?=w347:bool)
            n381 = And(x=w347, y=w348) -> (x .and. y?=w346:bool)
            n382 = case shown="True" w346 {
              frame False {
                n383 = local write "Active Trial"(FALSE ("Active_trial")) -> ()
              }
              frame True {
                n384 = shared-variable "My Computer\\michelle_library.lvlib\\Trial"() -> (w362:u32)  [unwired: 1 in, 1 out]
                n385 = local read "Stim_ID"() -> (w364:dbl[])
                n386 = Decrement(x=w362) -> (x-1=w363:u32)
                n387 = Index Array(array=w364, index=w363) -> (element=w361:dbl)
                n388 = case shown="1, Default" w361 {
                  frame 1, Default {
                    n389 = shared-variable "My Computer\\michelle_library.lvlib\\ISI_Time"() -> (w370:dbl)  [unwired: 1 in, 1 out]
                    n390 = local read "ActiveTime"() -> (w365:dbl)
                    n391 = Less?(x=w370, y=w365) -> (x < y?=w368:bool)
                    n392 = Greater?(x=w370, y=0.1) -> (0:w367:bool)
                    n393 = And(x=w368, y=w367) -> (x .and. y?=w366:bool)
                    n394 = case shown="True" w366 {
                      frame False {
                        n395 = local write "Active Trial"(FALSE ("Active Trial")) -> ()
                      }
                      frame True {
                        n396 = local read "Time"() -> (w374:dbl)
                        n397 = local write "Active Trial"(TRUE ("Active Trial")) -> ()
                        n398 = Add(x=w374, y=-0.11) -> (x+y=w372:dbl)
                        n399 = local write "Time of last lick"(w372) -> ()
                      }
                    }
                  }
                  frame 2 {
                    n400 = shared-variable "My Computer\\michelle_library.lvlib\\ISI_Time"() -> (w380:dbl)  [unwired: 1 in, 1 out]
                    n401 = local read "ActiveTime"() -> (w376:dbl)
                    n402 = Less?(x=w380, y=w376) -> (x < y?=w378:bool)
                    n403 = Greater?(x=w380, y=0.1) -> (0:w379:bool)
                    n404 = And(x=w379, y=w378) -> (x .and. y?=w377:bool)
                    n405 = case shown="True" w377 {
                      frame False {
                        n406 = local write "Active Trial"(FALSE ("Active Trial")) -> ()
                      }
                      frame True {
                        "Active Trial" <- TRUE ("Active Trial")
                      }
                    }
                  }
                }
              }
            }
            n407 = local read "Stop"() -> (w359:bool)
          }
        }
      }
    }
  }
